vi "FlexDDS-NG_AD9910_FormatSTP.vi"(8 "mirror frequency?":bool, 9 "phase degrees (0..360)":dbl, 10 "amplitude (0..1)":dbl=1.0, 11 "Frequency Hz (0)":dbl=10.0 format="%#_6f") -> (0 "phase offset word (POW) out":u16 format="%x", 1 "amplitude scale factor (ASF) out":u16=16383 format="%x", 2 "frequency tuning word (FTW) out":u32=42949673 format="%x", 3 "single-tone profile (STP) out":u64=4611404543493626921 format="%x")   [LabVIEW 2016]
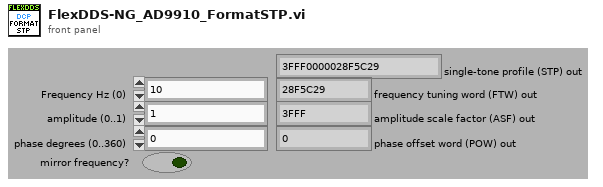
[diagram p1: front panel]
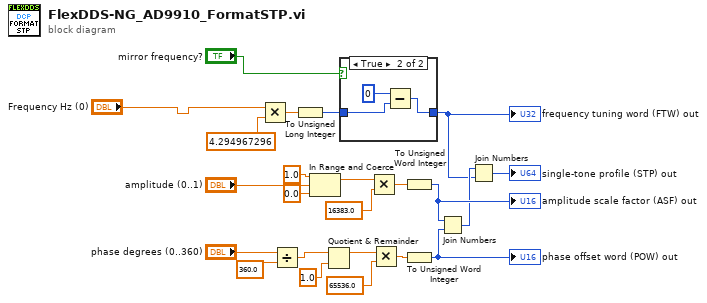
[diagram p0: block diagram]
diagram:
  n1 = Multiply(x="Frequency Hz (0)", y=4.294967296) -> (x*y=w14:dbl)
  n2 = Divide(x="phase degrees (0..360)", y=360.0) -> (x/y=w10:dbl)
  n3 = To Unsigned Long Integer(number=w14) -> (unsigned 32bit integer=w8:u32)
  n4 = In Range and Coerce(upper limit=1.0, x="amplitude (0..1)", lower limit=0.0) -> (coerced(x)=w19:dbl)  [unwired: 1 out]
  n5 = Quotient & Remainder(x=w10, y=1.0) -> (x-y*floor(x/y)=w21:dbl)  [unwired: 1 out]
  n6 = case shown="True" "mirror frequency?" {
    tunnel: w8 -> [w24 w26]
    tunnel: [w24 w25] -> w2
    frame False {
    }
    frame True {
      n7 = Subtract(x=u32 0 ("unsigned 32bit integer"), y=w26) -> (x-y=w25:u32)
    }
  }
  "frequency tuning word (FTW) out" <- w2
  n8 = Multiply(x=w19, y=16383.0) -> (x*y=w17:dbl)
  n9 = Multiply(x=w21, y=65536.0) -> (x*y=w16:dbl)
  n10 = To Unsigned Word Integer(number=w17) -> (unsigned 16bit integer=w6:u16)
  "amplitude scale factor (ASF) out" <- w6
  n11 = To Unsigned Word Integer(number=w16) -> (unsigned 16bit integer=w5:u16)
  "phase offset word (POW) out" <- w5
  n12 = Join Numbers(hi=w6, lo=w5) -> ((hi.lo)=w3:u32)
  n13 = Join Numbers(hi=w3, lo=w2) -> ((hi.lo)=→"single-tone profile (STP) out":u64)
